vi "LidarTestFilter.vi"() -> ()   [LabVIEW 2017]
uses:
  040-typeDefs/LidarPoint.ctl
panel:
  in  "stop":bool
  out "3 random points 2":T1
  in  "Point1":cluster{"X1":dbl, "Y1":dbl}
  in  "3 random points":T1
  out "XYflipped":T2[](array[typedef])
  out "XY Graph":cluster{dbl[], dbl[]}[](graph)
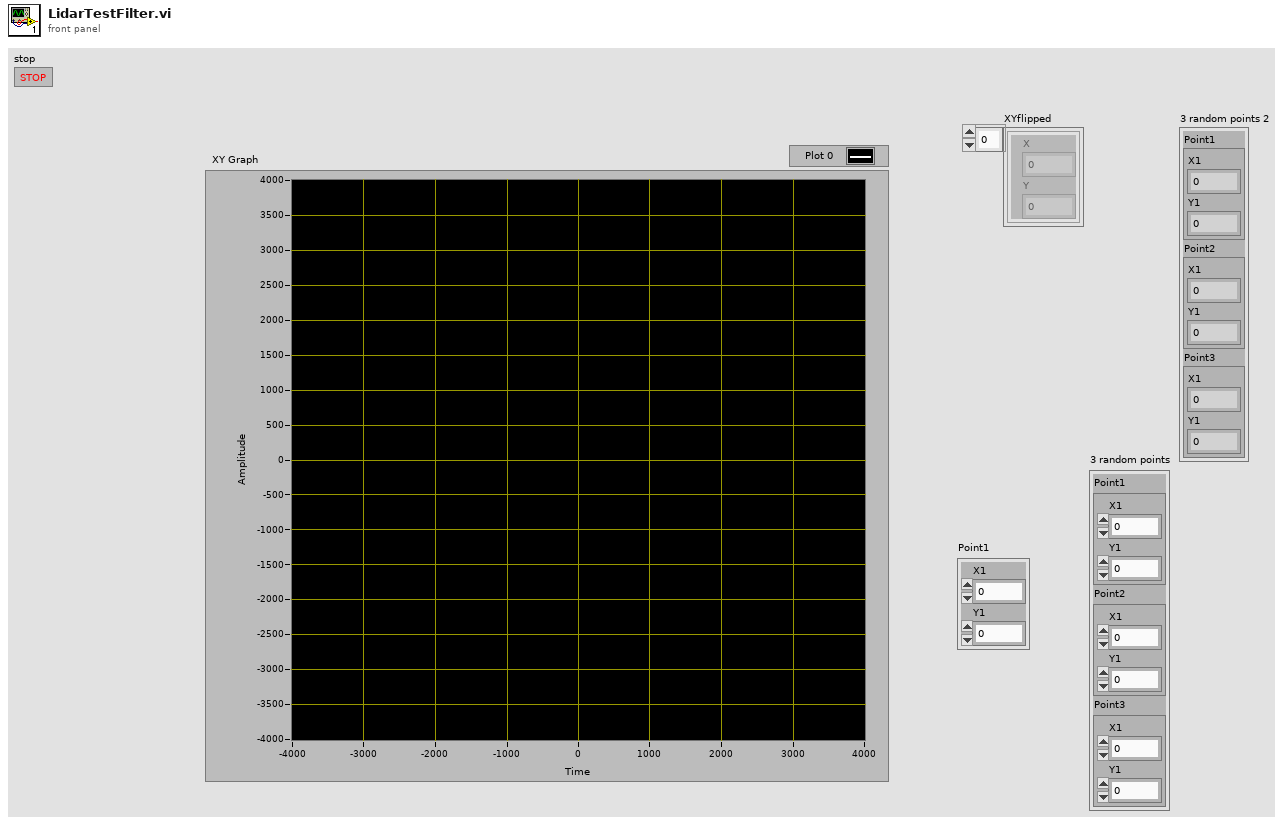
[diagram p1: front panel]
types:
  T1 = cluster{"Point1":cluster{"X1":dbl, "Y1":dbl}, "Point2":cluster{"X1":dbl, "Y1":dbl}, "Point3":cluster{"X1":dbl, "Y1":dbl}}
  T2 = typedef "LidarPoint.ctl" = cluster{"X":dbl, "Y":dbl}
  T3 = cluster{"Point1":cluster{"X1":bool, "Y1":bool}, "Point2":cluster{"X1":bool, "Y1":bool}, "Point3":cluster{"X1":bool, "Y1":bool}}
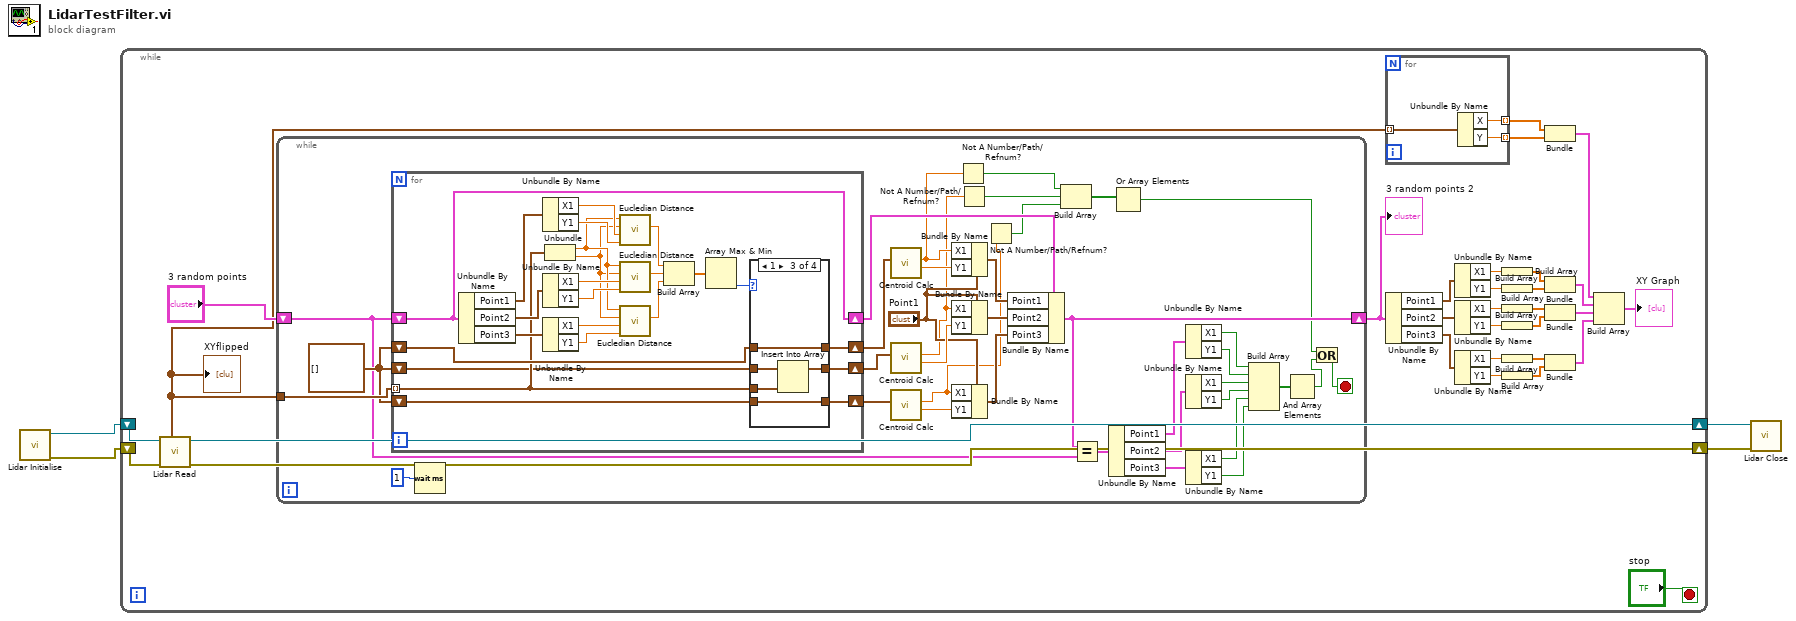
[diagram p0: block diagram]
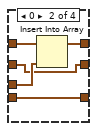
[diagram p3: hidden frame]
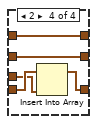
[diagram p4: hidden frame]
diagram:
  n1 = call "Lidar Initialise.vi"() -> ("error out"=w2:errorcluster, "VISA resource name out"=w4:refnum<visa-resource-name>)  [unwired: 10 in]
  n2 = while {
    shift-right: [w33] -> w3
    shift-left: w4 -> [w34]
    shift-right: [w31] -> w1
    shift-left: w2 -> [w32]
    stop <- "stop" stop-if-true
    n3 = call "Lidar Read.vi"("error in (no error)"=w32, "VISA resource name"=w34) -> ("error out"=w31:errorcluster, "VISA resource name out"=w33:refnum<visa-resource-name>, "XYflipped"=w5:T2[])  [unwired: 2 in, 4 out]
    "XYflipped" <- w5
    n4 = while {
      tunnel: w5 -> [w71]
      shift-right: [w58] -> w27
      shift-left: "3 random points" -> [w57]
      stop <- w37 stop-if-true
      w70 = T2[] []
      n5 = for {
        tunnel: w71 -> [w78] mode=indexing
        shift-right: [w75] -> w69
        shift-left: w70 -> [w79]
        shift-right: [w76] -> w68
        shift-left: w70 -> [w77]
        shift-right: [w73] -> w67
        shift-left: w70 -> [w74]
        shift-right: [w72] -> w66
        shift-left: w57 -> [w72]
        n6 = Unbundle By Name(w72) -> ("Point1"=w95:cluster{"X1":dbl, "Y1":dbl}, "Point2"=w94:cluster{"X1":dbl, "Y1":dbl}, "Point3"=w93:cluster{"X1":dbl, "Y1":dbl})
        n7 = Unbundle By Name(w95) -> ("X1"=w92:dbl, "Y1"=w91:dbl)
        n8 = Unbundle By Name(w94) -> ("X1"=w90:dbl, "Y1"=w89:dbl)
        n9 = Unbundle By Name(w93) -> ("X1"=w86:dbl, "Y1"=w85:dbl)
        n10 = Unbundle(w78) -> ("X"=w88:dbl, "Y"=w87:dbl)
        n11 = call "Eucledian Distance.vi"("Y2"=w91, "X2"=w92, "Y"=w87, "X"=w88) -> ("Distance"=w84:dbl)  [unwired: 7 in]
        n12 = call "Eucledian Distance.vi"("Y2"=w89, "X2"=w90, "Y"=w87, "X"=w88) -> ("Distance"=w83:dbl)  [unwired: 7 in]
        n13 = call "Eucledian Distance.vi"("Y2"=w85, "X2"=w86, "Y"=w87, "X"=w88) -> ("Distance"=w82:dbl)  [unwired: 7 in]
        n14 = Build Array(w84, w83, w82) -> (w81:dbl[])
        n15 = Array Max & Min(array=w81) -> (min index (indices)=w80:i32)  [unwired: 3 out]
        n16 = case shown="1" w80 {
          tunnel: w79 -> [w98 w103 w105 w110]
          tunnel: w78 -> [_ w102 w107 w112]
          tunnel: w77 -> [w97 w100 w108 w109]
          tunnel: [w97 w100 w106 w109] -> w76
          tunnel: [w98 w101 w105 w110] -> w75
          tunnel: w74 -> [w96 w99 w104 w113]
          tunnel: [w96 w99 w104 w111] -> w73
          frame Default {
          }
          frame 0 {
            n17 = Insert Into Array(array=w103, new element=w102) -> (w101:T2[])  [unwired: 1 in]
          }
          frame 1 {
            n18 = Insert Into Array(array=w108, new element=w107) -> (w106:T2[])  [unwired: 1 in]
          }
          frame 2 {
            n19 = Insert Into Array(array=w113, new element=w112) -> (w111:T2[])  [unwired: 1 in]
          }
        }
      }
      n20 = Wait (ms)(milliseconds to wait=u32 1) -> ()  [unwired: 1 out]
      n21 = call "Centroid Calc.vi"("Array"=w69) -> ("Y Centroid"=w65:dbl, "X Centroid"=w44:dbl)  [unwired: 9 in]
      n22 = call "Centroid Calc.vi"("Array"=w68) -> ("Y Centroid"=w64:dbl, "X Centroid"=w43:dbl)  [unwired: 9 in]
      n23 = call "Centroid Calc.vi"("Array"=w67) -> ("Y Centroid"=w63:dbl, "X Centroid"=w42:dbl)  [unwired: 9 in]
      n24 = Bundle By Name(cluster="Point1", "X1"=w44, "Y1"=w65) -> (w62:cluster{"X1":dbl, "Y1":dbl})
      n25 = Bundle By Name(cluster="Point1", "X1"=w43, "Y1"=w64) -> (w61:cluster{"X1":dbl, "Y1":dbl})
      n26 = Bundle By Name(cluster="Point1", "X1"=w42, "Y1"=w63) -> (w60:cluster{"X1":dbl, "Y1":dbl})
      n27 = Not A Number/Path/Refnum?(number/path/refnum=w44) -> (NaN/Path/Refnum?=w41:bool)
      n28 = Not A Number/Path/Refnum?(number/path/refnum=w43) -> (NaN/Path/Refnum?=w40:bool)
      n29 = Not A Number/Path/Refnum?(number/path/refnum=w42) -> (NaN/Path/Refnum?=w39:bool)
      n30 = Bundle By Name(cluster=w66, "Point1"=w62, "Point2"=w61, "Point3"=w60) -> (w58:T1)
      n31 = Build Array(w41, w40, w39) -> (w38:bool[])
      n32 = Equal?(x=w58, y=w57) -> (x = y?=w56:T3)
      n33 = Unbundle By Name(w56) -> ("Point1"=w55:cluster{"X1":bool, "Y1":bool}, "Point2"=w54:cluster{"X1":bool, "Y1":bool}, "Point3"=w53:cluster{"X1":bool, "Y1":bool})
      n34 = Or Array Elements(Boolean array=w38) -> (logical OR=w35:bool)
      n35 = Unbundle By Name(w55) -> ("X1"=w52:bool, "Y1"=w51:bool)
      n36 = Unbundle By Name(w54) -> ("X1"=w50:bool, "Y1"=w49:bool)
      n37 = Unbundle By Name(w53) -> ("X1"=w48:bool, "Y1"=w47:bool)
      n38 = Build Array(w52, w51, w50, w49, w48, w47) -> (w46:bool[])
      n39 = And Array Elements(Boolean array=w46) -> (logical AND=w36:bool)
      n40 = Or(x=w35, y=w36) -> (x .or. y?=w37:bool)
    }
    "3 random points 2" <- w27
    n41 = for {
      tunnel: w5 -> [w116] mode=indexing
      tunnel: [w115] -> w29 mode=indexing
      tunnel: [w114] -> w30 mode=indexing
      n42 = Unbundle By Name(w116) -> ("X"=w115:dbl, "Y"=w114:dbl)
    }
    n43 = Unbundle By Name(w27) -> ("Point1"=w26:cluster{"X1":dbl, "Y1":dbl}, "Point2"=w25:cluster{"X1":dbl, "Y1":dbl}, "Point3"=w24:cluster{"X1":dbl, "Y1":dbl})
    n44 = Unbundle By Name(w26) -> ("X1"=w23:dbl, "Y1"=w22:dbl)
    n45 = Unbundle By Name(w25) -> ("X1"=w21:dbl, "Y1"=w20:dbl)
    n46 = Unbundle By Name(w24) -> ("X1"=w19:dbl, "Y1"=w12:dbl)
    n47 = Build Array(w23) -> (w18:dbl[])
    n48 = Build Array(w22) -> (w17:dbl[])
    n49 = Build Array(w21) -> (w16:dbl[])
    n50 = Build Array(w20) -> (w15:dbl[])
    n51 = Build Array(w19) -> (w14:dbl[])
    n52 = Build Array(w12) -> (w13:dbl[])
    n53 = Bundle(w29, w30) -> (w8:cluster{dbl[], dbl[]})  [unwired: 1 in]
    n54 = Bundle(w18, w17) -> (w11:cluster{dbl[], dbl[]})  [unwired: 1 in]
    n55 = Bundle(w16, w15) -> (w10:cluster{dbl[], dbl[]})  [unwired: 1 in]
    n56 = Bundle(w14, w13) -> (w9:cluster{dbl[], dbl[]})  [unwired: 1 in]
    n57 = Build Array(w8, w11, w10, w9) -> (→"XY Graph":cluster{dbl[], dbl[]}[])
  }
  n58 = call "Lidar Close.vi"("error in (no error)"=w1, "VISA resource name"=w3) -> ()  [unwired: 9 in, 1 out]
